vi "Excel Export.vi"(0 "template Path":path=path "C:/Users/L025200.LUXSHARE/Desktop/Released VNA Automatic 20150329/Templete/QSFP+_IBM.xls", 1 "Data Basic Path":path=path "S:/PNA_DATA/QSFP+  IBM 3m/Sample_#1_150331", 2 "File Name List":string[](array[string]), 3 "Sheet Index List":i32[](array[numeric])=[1, 2, 3], 4 "Report Inf":string[](array[string]), 5 "Inf start":cluster{"row":i32, "column":i32}[](array[cluster])=[{"row"=2, "column"=0}, {"row"=2, "column"=0}, {"row"=2, "column"=0}], 6 "Sheet start(0,0)":cluster{"row":i32, "column":i32}[](array[cluster])=[{"row"=2, "column"=0}, {"row"=2, "column"=0}, {"row"=2, "column"=0}], 7 "error in (no error)":errorcluster caption="错误输入（无错误）", 8 "Demo":bool, 9 "Report Type":u16(ring) items=["Excel", "Excel&PDF"], 10 "reportSavePath":path, 11 "StartPage":i32=1, 13 "EndPage":i32=3) -> (12 "reportPath":path)   [LabVIEW 2011]
uses:
  <vilib>/addons/_office/_exclsub.llb/font.ctl
  <vilib>/Utility/NIReport.llb/NI_report.lvclass
  <vilib>/addons/_office/excel.llb/Excel Easy Table (str).vi
  <vilib>/Utility/file.llb/Read From Spreadsheet File (DBL).vi
  <vilib>/addons/_office/excel.llb/Excel Easy Table (num).vi
  <vilib>/Utility/NIReport.llb/Excel/NI_Excel.lvclass
  <vilib>/addons/_office/NI_ReportGenerationToolkit.lvlib
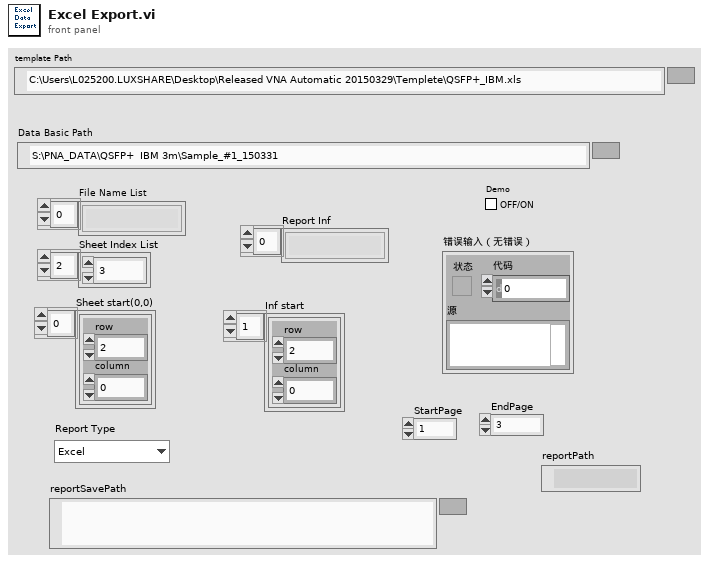
[diagram p1: front panel]
types:
  T1 = enum16{"Standard Report", "HTML", "Word", "Excel"}
  T2 = typedef "NI_ReportGenerationToolkit.lvlib/font.ctl" = cluster{"font name":string, "font size":dbl, "bold":u16, "italic":u16, "underline":u16, "strike through":u16, "font color":u32}
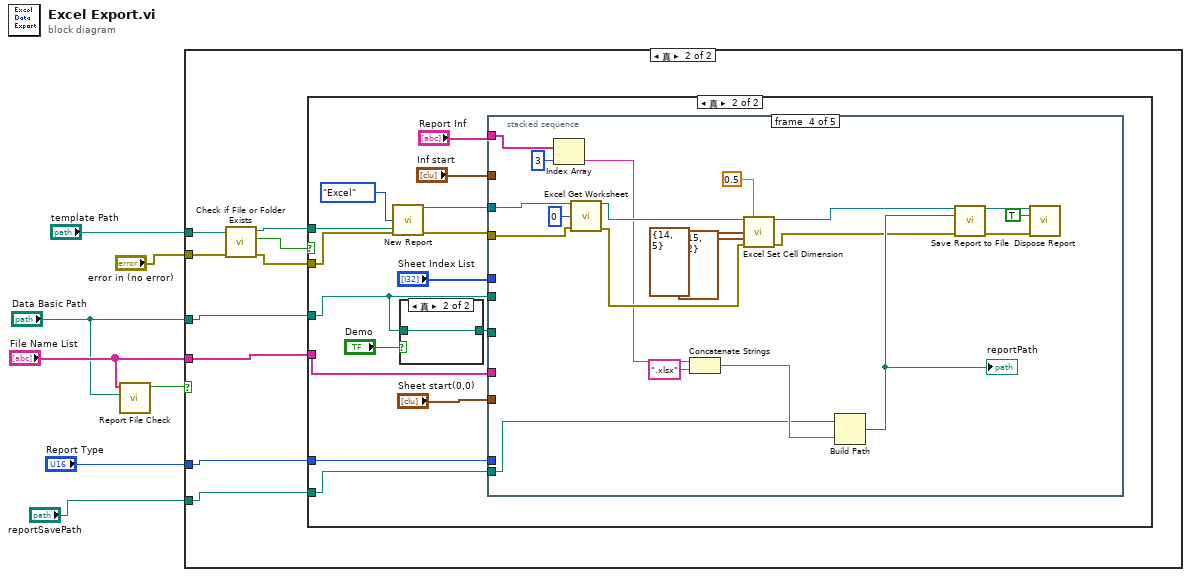
[diagram p0: block diagram]
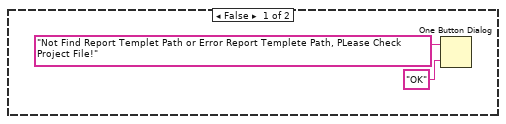
[diagram p3: hidden frame]
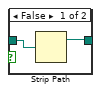
[diagram p4: hidden frame]
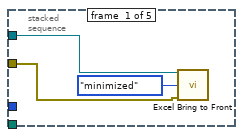
[diagram p5: hidden frame]
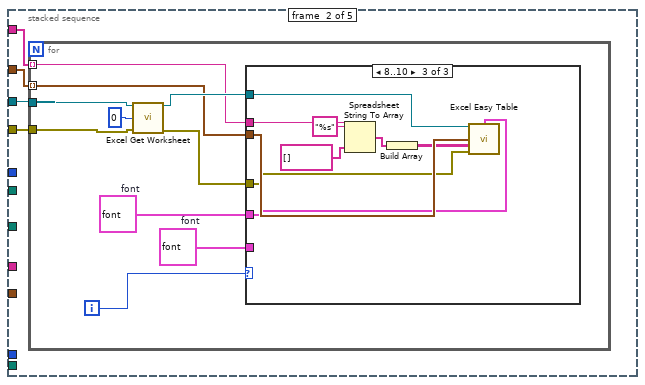
[diagram p6: hidden frame]
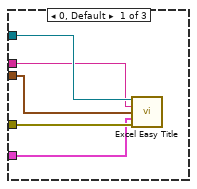
[diagram p7: hidden frame]
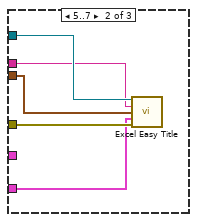
[diagram p8: hidden frame]
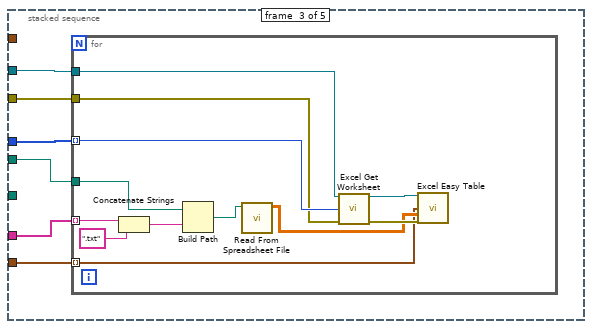
[diagram p9: hidden frame]
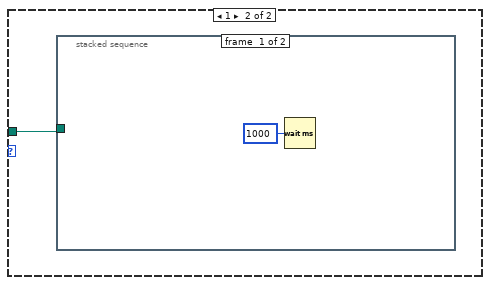
[diagram p11: hidden frame]
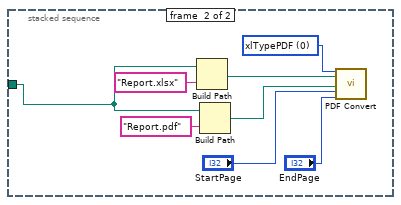
[diagram p12: hidden frame]
diagram:
  n1 = call "Report File Check.vi"("Data Basic Path"="Data Basic Path", "File Name List"="File Name List") -> ("OK?"=w3:bool)  [unwired: 9 in]
  n2 = case shown="真" w3 {
    tunnel: "File Name List" -> [_ w16]
    tunnel: "Data Basic Path" -> [_ w15]
    tunnel: "template Path" -> [_ w13]
    tunnel: "Report Type" -> [_ w14]
    tunnel: "error in (no error)" -> [_ w9]
    tunnel: "reportSavePath" -> [_ w8]
    frame False {
    }
    frame True {
      n3 = call <vilib>:"Check if File or Folder Exists.vi"("error in (no error)"=w9, "path"=w13) -> ("error out"=w10:errorcluster, "file or folder exists?"=w12:bool, "dup path"=w11:path)  [unwired: 7 in]
      n4 = case shown="真" w12 {
        tunnel: w16 -> [_ w32]
        tunnel: w15 -> [_ w21]
        tunnel: w11 -> [_ w25]
        tunnel: w14 -> [_ w24]
        tunnel: w10 -> [_ w23]
        tunnel: w8 -> [_ w19]
        frame False {
          n5 = One Button Dialog(message="Not Find Report Templet Path or Error Report Templete Path, PLease Check Project File!" ("消息"), button name ("OK")="OK" ("按钮名称（“确定”）")) -> ()  [unwired: 1 out]
        }
        frame True {
          n6 = call <vilib>:"New Report.vi"("report type"=T1."Excel", "template (empty)"=w25, "error in (no error)"=w23) -> ("report out"=w30:refnum<class "NI_report.lvclass">, "error out"=w28:errorcluster)  [unwired: 11 in]
          n7 = case shown="真" "Demo" {
            tunnel: w21 -> [w35 w36]
            tunnel: [w34 w36] -> w20
            frame False {
              n8 = Strip Path(path=w35) -> (stripped path=w34:path)  [unwired: 1 out]
            }
            frame True {
            }
          }
          n9 = stacked-sequence {
            tunnel: w32 -> [_ _ w78 _ _]
            tunnel: w21 -> [_ _ w77 _ _]
            tunnel: "Sheet Index List" -> [_ _ w76 _ _]
            tunnel: w30 -> [w38 w43 w75 w110 _]
            tunnel: "Sheet start(0,0)" -> [_ _ w74 _ _]
            tunnel: w28 -> [w37 w42 w73 w105 _]
            tunnel: "Report Inf" -> [_ w41 _ w96 _]
            tunnel: "Inf start" -> [_ w40 _ _ _]
            tunnel: w24 -> [_ _ _ _ w112]
            tunnel: w20 -> [_ _ _ _ w111]
            tunnel: w19 -> [_ _ _ w91 _]
            frame #0 {
              n10 = call <vilib>:"Excel Bring to Front.vi"("report in"=w38, "window state (maximized)"=enum16{"maximized", "minimized", "normal"}."minimized", "error in (no error)"=w37) -> ()  [unwired: 11 in, 2 out]
            }
            frame #1 {
              n11 = for {
                tunnel: w43 -> [w53]
                tunnel: w42 -> [w52]
                tunnel: w41 -> [w48] mode=indexing
                tunnel: w40 -> [w47] mode=indexing
                i -> [w50]
                w44 = T2 {"font name"="Arial", "font size"=16.0, "bold"=2, "italic"=0, "underline"=0, "strike through"=0, "font color"=16777216}  # font
                w45 = T2 {"font name"="Arial", "font size"=10.0, "bold"=2, "italic"=0, "underline"=0, "strike through"=0, "font color"=16777216}  # font
                n12 = call <vilib>:"Excel Get Worksheet.vi"("report in"=w53, "worksheet index (0)"=0, "error in (no error)"=w52) -> ("report out"=w49:refnum<class "NI_report.lvclass">, "error out"=w46:errorcluster)  [unwired: 11 in]
                n13 = case shown="8..10" w50 {
                  tunnel: w49 -> [w58 w63 w70]
                  tunnel: w48 -> [w57 w62 w72]
                  tunnel: w47 -> [w56 w61 w69]
                  tunnel: w46 -> [w55 w60 w68]
                  tunnel: w45 -> [w54 _ w64]
                  tunnel: w44 -> [_ w59 _]
                  frame 0, Default {
                    n14 = call <vilib>:"Excel Easy Title.vi"("report in"=w58, "title"=w57, "start (0, 0)"=w56, "font"=w54, "error in (no error)"=w55) -> ()  [unwired: 8 in, 3 out]
                  }
                  frame 5..7 {
                    n15 = call <vilib>:"Excel Easy Title.vi"("report in"=w63, "title"=w62, "start (0, 0)"=w61, "font"=w59, "error in (no error)"=w60) -> ()  [unwired: 8 in, 3 out]
                  }
                  frame 8..10 {
                    n16 = Spreadsheet String To Array(format string="%s" ("格式字符串"), spreadsheet string=w72, array type (2D Dbl)=string[] [] ("添加的数组")) -> (array=w66:string[])  [unwired: 1 in]
                    n17 = Build Array(w66) -> (w65:string[][])
                    n18 = call-poly <vilib>:"Excel Easy Table.vi"("report in"=w70, "font"=w64, "start (0, 0)"=w69, "text data"=w65, "error in (no error)"=w68) -> ()  [unwired: 6 in, 5 out]
                  }
                }
              }
            }
            frame #2 {
              n19 = for {
                tunnel: w78 -> [w90] mode=indexing
                tunnel: w77 -> [w87]
                tunnel: w76 -> [w82] mode=indexing
                tunnel: w75 -> [w83]
                tunnel: w74 -> [w80] mode=indexing
                tunnel: w73 -> [w79]
                n20 = Concatenate Strings(w90, ".txt" ("字符串")) -> (w89:string)
                n21 = Build Path(base path=w87, name or relative path=w89) -> (appended path=w86:path)
                n22 = call-poly <vilib>:"Read From Spreadsheet File.vi"("file path (dialog if empty)"=w86) -> ("all rows"=w81:dbl[][])  [unwired: 6 in, 4 out]
                n23 = call <vilib>:"Excel Get Worksheet.vi"("report in"=w83, "worksheet index (0)"=w82, "error in (no error)"=w79) -> ("report out"=w84:refnum<class "NI_report.lvclass">, "error out"=w85:errorcluster)  [unwired: 11 in]
                n24 = call-poly <vilib>:"Excel Easy Table.vi"("report in"=w84, "start (0, 0)"=w80, "text data"=w81, "error in (no error)"=w85) -> ()  [unwired: 7 in, 5 out]
              }
            }
            frame #3 {
              n25 = Index Array(array=w96, index=3 ("索引")) -> (element=w94:string)
              n26 = call <vilib>:"Excel Get Worksheet.vi"("report in"=w110, "worksheet index (0)"=0, "error in (no error)"=w105) -> ("report out"=w100:refnum<class "NI_report.lvclass">, "error out"=w98:errorcluster)  [unwired: 11 in]
              n27 = Concatenate Strings(w94, ".xlsx" ("字符串")) -> (w92:string)
              n28 = call <vilib>:"Excel Set Cell Dimension.vi"("report in"=w100, "width (-1)"=0.5, "start (-1, -1)"=cluster{"row":i32, "column":i32} {"row"=14, "column"=5}, "end (-1, -1)"=cluster{"row":i32, "column":i32} {"row"=15, "column"=12}, "error in (no error)"=w98) -> ("report out"=w99:refnum<class "NI_report.lvclass">, "error out"=w97:errorcluster)  [unwired: 9 in]
              n29 = Build Path(base path=w91, name or relative path=w92) -> (appended path=w104:path)
              "reportPath" <- w104
              n30 = call-dynamic "Save Report to File.vi"("report in"=w99, "report file path"=w104, "error in (no error)"=w97) -> ("report out"=w107:refnum<class "NI_report.lvclass">, "error out"=w108:errorcluster)  [unwired: 11 in]
              n31 = call-dynamic "Dispose Report.vi"("report in"=w107, "wait until printing completed? (T)"=TRUE, "error in (no error)"=w108) -> ()  [unwired: 12 in, 1 out]
            }
            frame #4 {
              n32 = case shown="0, 默认" w112 {
                tunnel: w111 -> [_ w113]
                frame 0, Default {
                }
                frame 1 {
                  n33 = stacked-sequence {
                    tunnel: w113 -> [_ w115]
                    frame #0 {
                      n34 = Wait (ms)(milliseconds to wait=u32 1000 ("等待时间（毫秒）")) -> ()  [unwired: 1 out]
                    }
                    frame #1 {
                      w118 = 0 items=["xlTypePDF", "xlTypeXPS"] ("Type")
                      n35 = Build Path(base path=w115, name or relative path="Report.xlsx" ("名称或相对路径")) -> (appended path=w120:path)
                      n36 = Build Path(base path=w115, name or relative path="Report.pdf" ("名称或相对路径")) -> (appended path=w119:path)
                      n37 = call "PDF Convert.vi"("Type"=w118, "Excel Report Path"=w120, "PDF  Report Target Path"=w119, "StartPage"="StartPage", "EndPage"="EndPage") -> ()  [unwired: 15 in]
                    }
                  }
                }
              }
            }
          }
        }
      }
    }
  }
